vi "Write Linker Info to File.vi"(6 "New Names":string[](array[string]), 8 "error in (no error)":errorcluster, 9 "Old Names":string[](array[string]), 10 "new paths":path[](array[path]), 11 "files to change":path[](array[path])) -> (0 "error out":errorcluster)   [LabVIEW 2020, in "Save for Previous Version.lvlib"]
uses:
  Save for Previous Version.lvlib
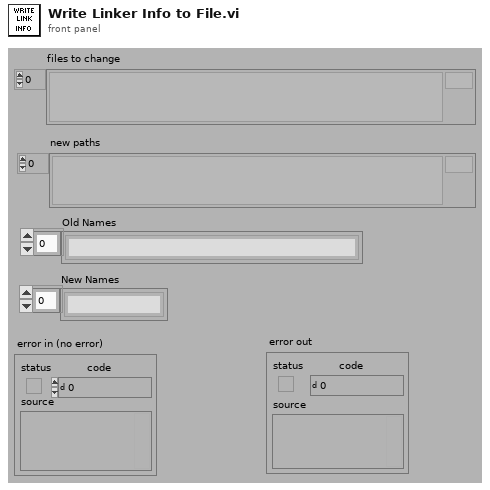
[diagram p1: front panel]
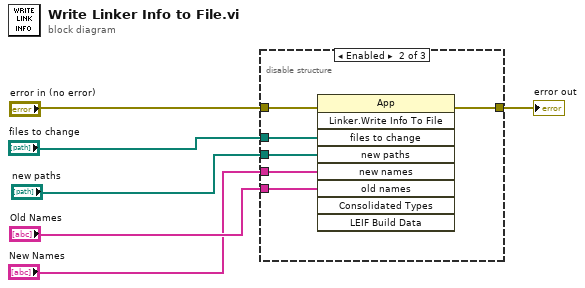
[diagram p0: block diagram]
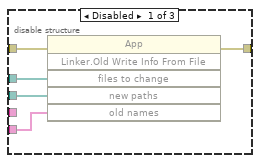
[diagram p2: hidden frame]
diagram:
  n1 = disable-structure shown="Enabled" {
    disable-tunnel: "files to change" -> [w11 w17 _]
    disable-tunnel: "new paths" -> [w10 w16 _]
    disable-tunnel: [w9 w15 _] -> w4
    disable-tunnel: "error in (no error)" -> [w8 w14 _]
    disable-tunnel: "Old Names" -> [w7 w12 _]
    disable-tunnel: "New Names" -> [_ w13 _]
    frame Disabled {
      n2 = invoke class="App" method="Linker.Old Write Info From File"(error in=w8, "files to change"=w11, "new paths"=w10, "old names"=w7) -> (error out=w9:errorcluster)  [unwired: 2 in, 5 out]
    }
    frame Enabled {
      n3 = invoke class="App" method="Linker.Write Info To File"(error in=w14, "files to change"=w17, "new paths"=w16, "new names"=w13, "old names"=w12) -> (error out=w15:errorcluster)  [unwired: 4 in, 8 out]
    }
    frame Disabled {
    }
  }
  "error out" <- w4
